vi "VisionAlign.vi"(8 "Error In":errorcluster, 11 "Control Mode":enum16{"Boiler", "Peg"}(ring)) -> (0 "Error Out":errorcluster)   [LabVIEW 2017]
uses:
  <vilib>/addons/control/pid/NI_PID_pid.lvlib
  <vilib>/Rock Robotics/Network Tables/NT Read Number.vi
  Robot Global Data.vi
  <vilib>/addons/control/pid/pid.llb/PID (DBL).vi
panel:
  out "Drive Multiplier":dbl
  out "Offset":dbl
  out "Setpoint":dbl
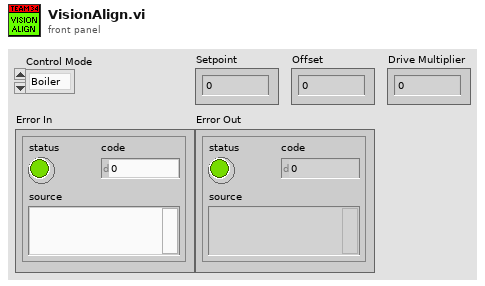
[diagram p1: front panel]
types:
  T1 = cluster{"proportional gain (Kc)":dbl, "integral time (Ti, min)":dbl, "derivative time (Td, min)":dbl}
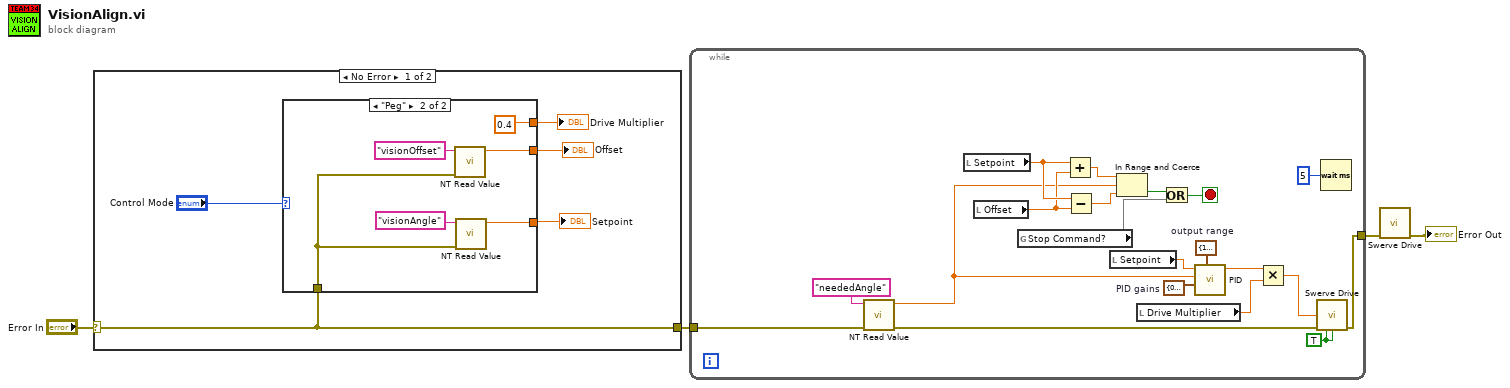
[diagram p0: block diagram]
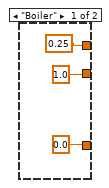
[diagram p2: hidden frame]
diagram:
  n1 = case shown="No Error" "Error In" {
    selector: "Error In" -> [w5 w19]
    tunnel: [w5 w19] -> w1
    frame No Error {
      n2 = case shown="\"Peg\"" "Control Mode" {
        tunnel: [0.25 0.4] -> w7
        tunnel: [1.0 ("Numeric") w15] -> w8
        tunnel: [0.0 ("Numeric") w14] -> w9
        tunnel: w5 -> [_ w13]
        frame "Boiler" {
        }
        frame "Peg" {
          n3 = call-poly <vilib>:"NT Read Value.vi"("error in"=w13, "Name"="visionOffset") -> ("Numeric"=w15:dbl)  [unwired: 8 in, 1 out]
          n4 = call-poly <vilib>:"NT Read Value.vi"("error in"=w13, "Name"="visionAngle") -> ("Numeric"=w14:dbl)  [unwired: 8 in, 1 out]
        }
      }
      "Drive Multiplier" <- w7
      "Setpoint" <- w9
      "Offset" <- w8
    }
    frame Error {
    }
  }
  n5 = while {
    tunnel: [w28] -> w4
    tunnel: w1 -> [w37]
    stop <- w36 stop-if-true
    w29 = cluster{"output high":dbl, "output low":dbl} {"output high"=1.0, "output low"=-1.0}  # output range
    w30 = T1 {"proportional gain (Kc)"=0.04, "integral time (Ti, min)"=0.0, "derivative time (Td, min)"=0.0}  # PID gains
    w31 = TRUE ("Robot Centric?")
    n6 = call-poly <vilib>:"NT Read Value.vi"("error in"=w37, "Name"="neededAngle") -> ("error out"=w20:errorcluster, "Numeric"=w22:dbl)  [unwired: 8 in]
    n7 = local read "Setpoint"() -> (w25:dbl)
    n8 = local read "Offset"() -> (w24:dbl)
    n9 = global read "Robot Global Data.vi" "Stop Command?"() -> (w34)
    n10 = Add(x=w25, y=w24) -> (x+y=w33:dbl)
    n11 = Subtract(x=w25, y=w24) -> (x-y=w32:dbl)
    n12 = local read "Setpoint"() -> (w23:dbl)
    n13 = In Range and Coerce(upper limit=w33, x=w22, lower limit=w32) -> (In Range?=w35:bool)  [unwired: 1 out]
    n14 = local read "Drive Multiplier"() -> (w27:dbl)
    n15 = Or(x=w35, y=w34) -> (x .or. y?=w36:bool)
    n16 = call-poly <vilib>:"PID.vi"("output range"=w29, "PID gains"=w30, "process variable"=w22, "setpoint"=w23) -> ("output"=w26:dbl)  [unwired: 6 in, 1 out]
    n17 = Multiply(x=w26, y=w27) -> (x*y=w21:dbl)
    n18 = call "Swerve Drive.vi"("Z"=w21, "Error In"=w20, "Robot Centric?"=w31, "Autonomous?"=w31) -> ("Error Out"=w28:errorcluster)  [unwired: 7 in, 4 out]
    n19 = Wait (ms)(milliseconds to wait=u32 5) -> ()  [unwired: 1 out]
  }
  n20 = call "Swerve Drive.vi"("Error In"=w4) -> ("Error Out"=→"Error Out":errorcluster)  [unwired: 10 in, 4 out]
